vi "Pair with Largest in Window.vi"(8 "error in (no error)":errorcluster, 10 "Allowed dt":dbl=0.1, 11 "State in":T1={"Raw File Data"="", "Deduplicated String Array"=[], "1-Entries"=[], "2-Entries"=[], "3-Entries"=[], "Bounds"={"M-Min"=0, "M-Max"=1023, "S-Min"=0, "S-Max"=1023}, "Matched ADC Values - Nearest"=[], "Match Entry Indices - Nearest"=[], "Filtered 1-Entries"=[], "Filtered 2-Entries"=[], "Filtered 3-Entries"=[], "Total Duration"=0.0, "Matched ADC Values - Largest"=[], "Match Entry Indices - Largest"=[]}) -> (0 "error out":errorcluster, 3 "State out":T1={"Raw File Data"="", "Deduplicated String Array"=[], "1-Entries"=[], "2-Entries"=[], "3-Entries"=[], "Bounds"={"M-Min"=0, "M-Max"=1023, "S-Min"=0, "S-Max"=1023}, "Matched ADC Values - Nearest"=[], "Match Entry Indices - Nearest"=[], "Filtered 1-Entries"=[], "Filtered 2-Entries"=[], "Filtered 3-Entries"=[], "Total Duration"=0.0, "Matched ADC Values - Largest"=[], "Match Entry Indices - Largest"=[]})   [LabVIEW 2019, in "Muon Data Post-Processing.lvlib"]
uses:
  Muon Data Post-Processing.lvlib
  State Data.ctl
  File Entry.ctl
  ADC Bounds.ctl
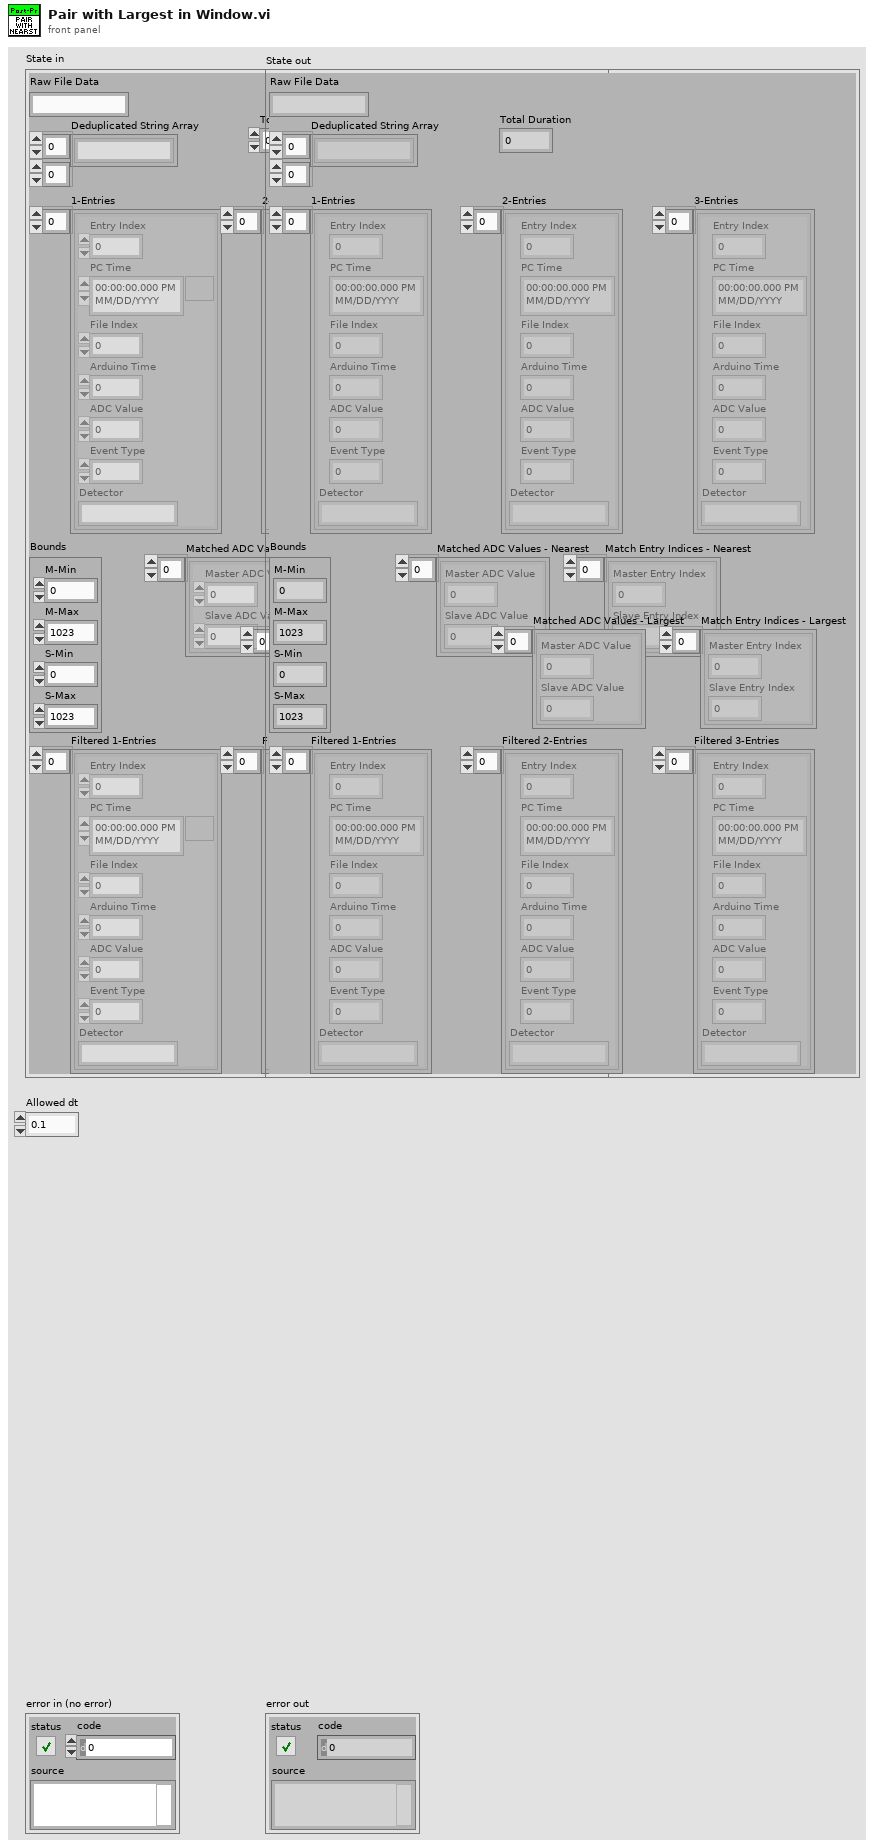
[diagram p1: front panel]
types:
  T1 = typedef "Muon Data Post-Processing.lvlib/State Data.ctl" = cluster{"Raw File Data":string, "Deduplicated String Array":string[][], "1-Entries":T2[], "2-Entries":T2[], "3-Entries":T2[], "Bounds":T3, "Matched ADC Values - Nearest":cluster{"Master ADC Value":i32, "Slave ADC Value":i32}[], "Match Entry Indices - Nearest":cluster{"Master Entry Index":i32, "Slave Entry Index":i32}[], "Filtered 1-Entries":T2[], "Filtered 2-Entries":T2[], "Filtered 3-Entries":T2[], "Total Duration":dbl, "Matched ADC Values - Largest":cluster{"Master ADC Value":i32, "Slave ADC Value":i32}[], "Match Entry Indices - Largest":cluster{"Master Entry Index":i32, "Slave Entry Index":i32}[]}
  T2 = typedef "Muon Data Post-Processing.lvlib/File Entry.ctl" = cluster{"Entry Index":i32, "PC Time":timestamp, "File Index":i32, "Arduino Time":i32, "ADC Value":i32, "Event Type":i32, "Detector":string}
  T3 = typedef "Muon Data Post-Processing.lvlib/ADC Bounds.ctl" = cluster{"M-Min":u16, "M-Max":u16, "S-Min":u16, "S-Max":u16}
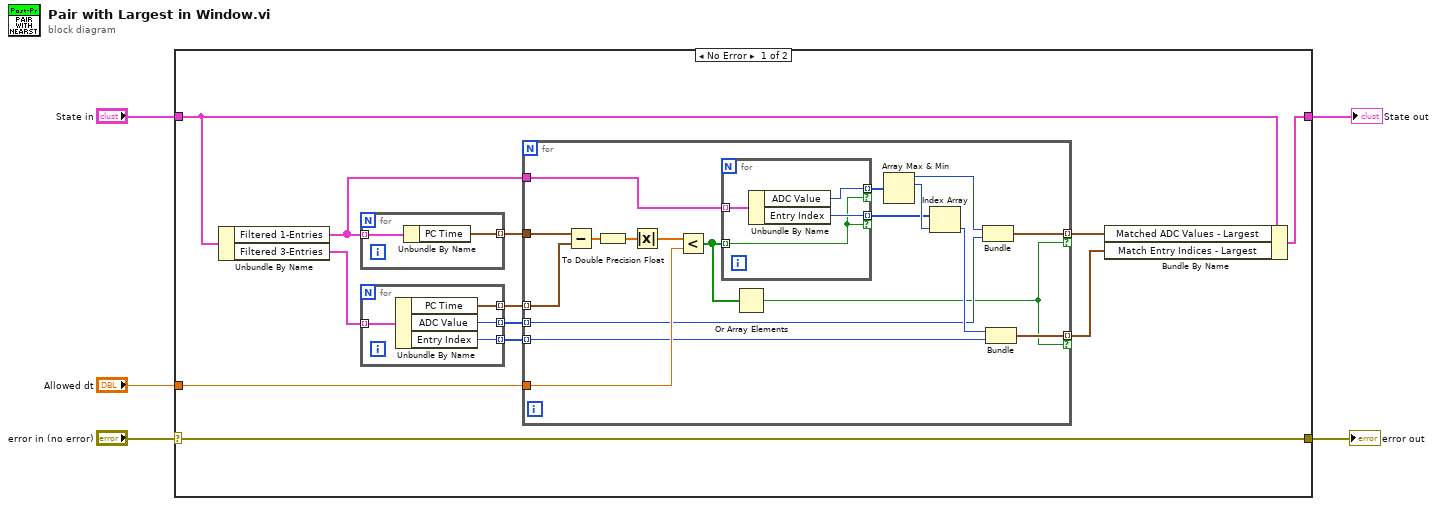
[diagram p0: block diagram]
diagram:
  n1 = case shown="No Error" "error in (no error)" {
    selector: "error in (no error)" -> [w16 w46]
    tunnel: [w13 w47] -> w4
    tunnel: "State in" -> [w17 w47]
    tunnel: [w16 w46] -> w2
    tunnel: "Allowed dt" -> [w11 _]
    frame No Error {
      n2 = Unbundle By Name(w17) -> ("Filtered 1-Entries"=w10:T2[], "Filtered 3-Entries"=w12:T2[])
      n3 = for {
        tunnel: w10 -> [w22] mode=indexing
        tunnel: [w23] -> w15 mode=indexing
        n4 = Unbundle By Name(w22) -> ("PC Time"=w23:timestamp)
      }
      n5 = for {
        tunnel: w12 -> [w20] mode=indexing
        tunnel: [w21] -> w14 mode=indexing
        tunnel: [w19] -> w7 mode=indexing
        tunnel: [w18] -> w6 mode=indexing
        n6 = Unbundle By Name(w20) -> ("PC Time"=w21:timestamp, "ADC Value"=w19:i32, "Entry Index"=w18:i32)
      }
      n7 = for {
        tunnel: w15 -> [w39]
        tunnel: w14 -> [w38] mode=indexing
        tunnel: w11 -> [w36]
        tunnel: w10 -> [w35]
        tunnel: [w30] -> w9 mode=indexing if=w24
        tunnel: [w28] -> w8 mode=indexing if=w24
        tunnel: w7 -> [w27] mode=indexing
        tunnel: w6 -> [w26] mode=indexing
        n8 = Subtract(x=w39, y=w38) -> (x-y=w41:dbl[])
        n9 = To Double Precision Float(number=w41) -> (double precision float=w40:dbl[])
        n10 = Absolute Value(x=w40) -> (abs(x)=w37:dbl[])
        n11 = Less?(x=w37, y=w36) -> (x < y?=w25:bool[])
        n12 = for {
          tunnel: w35 -> [w45] mode=indexing
          tunnel: w25 -> [w42] mode=indexing
          tunnel: [w44] -> w34 mode=indexing if=w42
          tunnel: [w43] -> w32 mode=indexing if=w42
          n13 = Unbundle By Name(w45) -> ("ADC Value"=w44:i32, "Entry Index"=w43:i32)
        }
        n14 = Or Array Elements(Boolean array=w25) -> (logical OR=w24:bool)
        n15 = Array Max & Min(array=w34) -> (max value=w31:i32, max index (indices)=w33:i32)  [unwired: 2 out]
        n16 = Index Array(array=w32, index=w33) -> (element=w29:i32)
        n17 = Bundle(w31, "ADC Value"=w27) -> (w30:cluster{i32, "ADC Value":i32})  [unwired: 1 in]
        n18 = Bundle("Entry Index"=w29, "Entry Index"=w26) -> (w28:cluster{"Entry Index":i32, "Entry Index":i32})  [unwired: 1 in]
      }
      n19 = Bundle By Name(cluster=w17, "Matched ADC Values - Largest"=w9, "Match Entry Indices - Largest"=w8) -> (w13:T1)
    }
    frame Error {
    }
  }
  "State out" <- w4
  "error out" <- w2
